vi "Datasheet Summarize Channel Data.vi"(1 "Channel Data":T1[](array[typedef])) -> (0 "HTM Table Rows":string)   [LabVIEW 2011]
uses:
  TDMS/TDMS Channel (Sxx).ctl
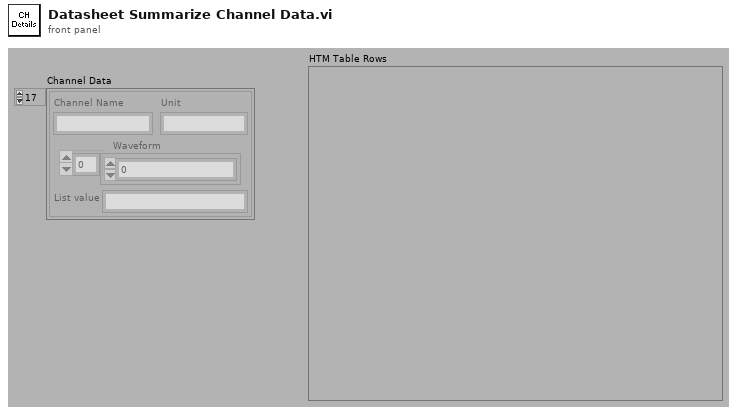
[diagram p1: front panel]
types:
  T1 = typedef "TDMS Channel (Sxx).ctl" = cluster{"Channel Name":string, "Waveform":dbl[], "Unit":string, "List value":string}
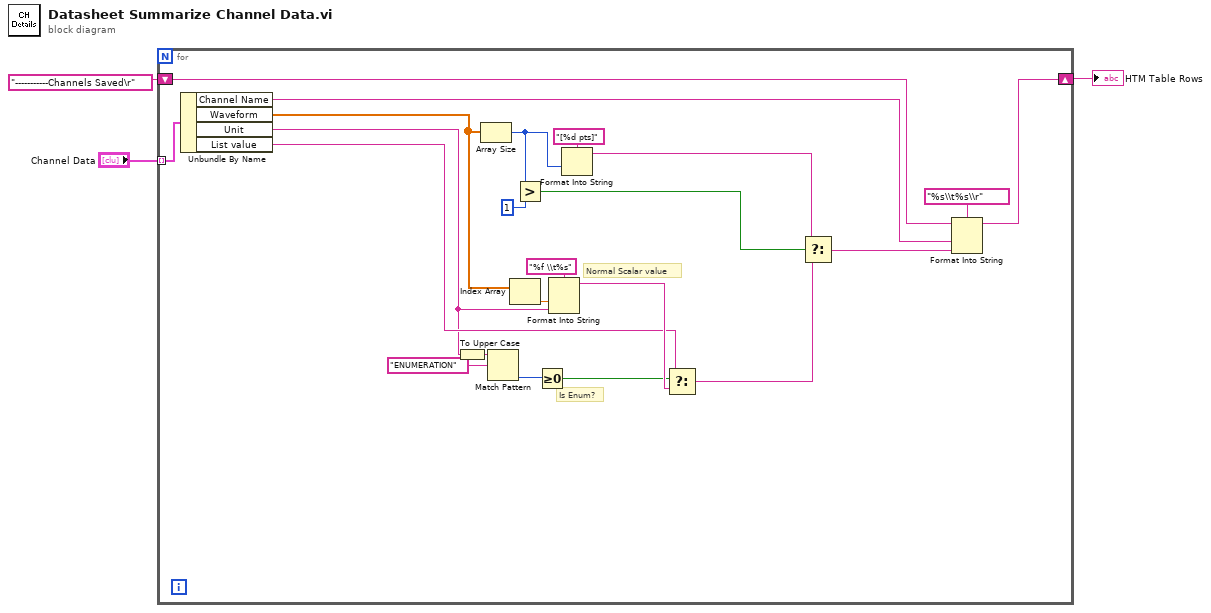
[diagram p0: block diagram]
diagram:
  n1 = for {
    shift-right: [w25] -> w3
    shift-left: "-----------Channels Saved\r" ("format string") -> [w24]
    tunnel: "Channel Data" -> [w23] mode=indexing
    # "Is Enum?"
    # "Normal Scalar value"
    n2 = Unbundle By Name(w23) -> ("Channel Name"=w21:string, "Waveform"=w20:dbl[], "Unit"=w8:string, "List value"=w9:string)
    n3 = To Upper Case(1:w8) -> (0:w10:string)
    n4 = Array Size(array=w20) -> (size(s)=w6:i32)
    n5 = Match Pattern(string=w10, regular expression="ENUMERATION" ("format string")) -> (offset past match=w13:i32)  [unwired: 4 out]
    n6 = Index Array(array=w20) -> (element=w15:dbl)  [unwired: 1 in]
    n7 = Greater?(x=w6, y=1) -> (0:w7:bool)
    n8 = Greater Or Equal To 0?(x=w13) -> (x >= 0?=w11:bool)
    n9 = Format Into String(format string="%f \\t%s", w15, w8) -> (resulting string=w12:string)  [unwired: 2 in, 1 out]
    n10 = Format Into String(format string="[%d pts]", w6) -> (resulting string=w17:string)  [unwired: 2 in, 1 out]
    n11 = Select(t=w9, s=w11, f=w12) -> (s? t:f=w5:string)
    n12 = Select(t=w17, s=w7, f=w5) -> (s? t:f=w22:string)
    n13 = Format Into String(format string="%s\\t%s\\r", initial string=w24, w21, w22) -> (resulting string=w25:string)  [unwired: 1 in, 1 out]
  }
  "HTM Table Rows" <- w3
